vi "Set Speaker Elapsed Time.vi"(8 "error in":errorcluster, 11 "PAS in":refnum<class "PAS.lvclass">=refnum) -> (0 "error out":errorcluster, 1 "maxElapsedTime":cluster{"true":dbl, "false":dbl}, 3 "PAS out":refnum<class "PAS.lvclass">)   [LabVIEW 2014, in "PAS.lvclass"]
doc: "Set the speakerr elapsed time (override to enable communication via chosen communication method of child class)."
uses:
  PAS.lvclass
  Switch/Switch.lvclass
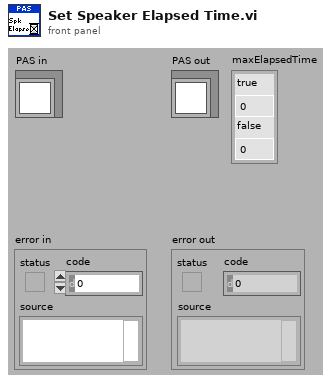
[diagram p1: front panel]
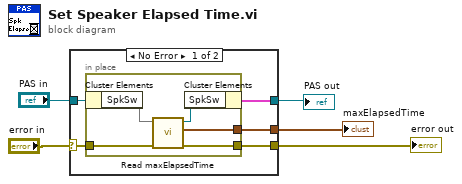
[diagram p0: block diagram]
diagram:
  n1 = case shown="No Error" "error in" {
    selector: "error in" -> [w6 w17]
    tunnel: [w7 w16] -> w4
    tunnel: [w10 _] -> w3
    tunnel: [w9 w17] -> w2
    tunnel: "PAS in" -> [w8 w16]
    frame No Error {
      n2 = in-place {
        in-place-border: [w15] -> w10
        in-place-border: [w14] -> w9
        in-place-border: w6 -> [w11]
        n3 = in-place-cluster #1(w8) -> ("SpkSw"=w13)
        n4 = call "Read maxElapsedTime.vi"("error in"=w11, "Switch in"=w13) -> ("error out"=w14:errorcluster, "maxElapsedTime"=w15:cluster{"Period":sgl, "Length":sgl}, "Switch out"=w12:refnum<class "Switch.lvclass">)  [unwired: 7 in]
        n5 = in-place-cluster #1("SpkSw"=w12) -> (w7:cluster{})
      }
    }
    frame Error {
    }
  }
  "PAS out" <- w4
  "maxElapsedTime" <- w3
  "error out" <- w2
